vi "G4SubTemplate_Singleton_6x8x6_Init.vi"(0 "reference in":refnum<class "G4SubTemplate_Singleton_6x8x6.lvclass"> caption="This control should only be used when\na sub class is inheriting this class", 5 "error in (no error)":errorcluster) -> (14 "reference out":refnum<class "G4SubTemplate_Singleton_6x8x6.lvclass"> caption="This indicator should only be used when\na sub class is inheriting this class", 19 "error out":errorcluster)   [LabVIEW 2014, in "G4SubTemplate_Singleton_6x8x6.lvclass"]
uses:
  <resource>/Framework/Providers/Open_GDS/ClassProviders/Provider_EndevoGOOP400/Templates/G4SubTemplate_Singleton_6x8x6/G4SubTemplate_Singleton_6x8x6.lvclass
  <resource>/Framework/Providers/Open_GDS/ClassProviders/Provider_EndevoGOOP400/Templates/G4BaseTemplate_Singleton_6x8x6/G4BaseTemplate_Singleton_6x8x6.lvclass
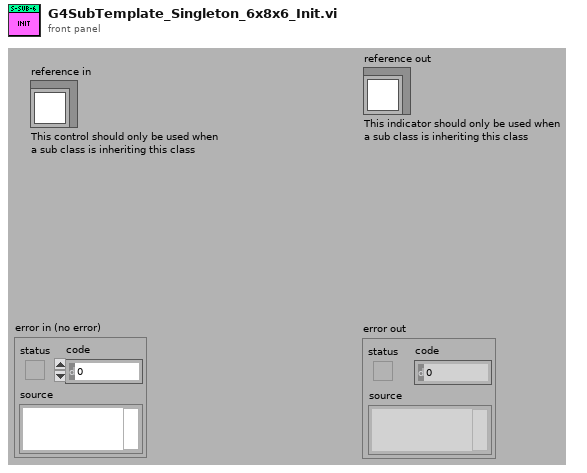
[diagram p1: front panel]
types:
  T1 = typedef "G4SubTemplate_Singleton_6x8x6.lvclass/ObjectAttributes.ctl" = cluster{"Attribute1":dbl}
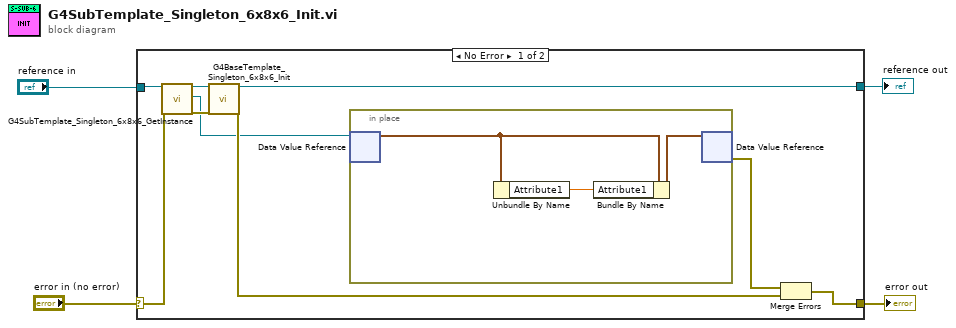
[diagram p0: block diagram]
diagram:
  n1 = case shown="No Error" "error in (no error)" {
    selector: "error in (no error)" -> [w10 w18]
    tunnel: [w12 w18] -> w3
    tunnel: "reference in" -> [w8 w17]
    tunnel: [w7 w17] -> w1
    frame No Error {
      n2 = call <resource>:"G4SubTemplate_Singleton_6x8x6_GetInstance.vi"("reference in"=w8, "error in (no error)"=w10) -> ("reference out"=w6:refnum<class "G4SubTemplate_Singleton_6x8x6.lvclass">, "DVRRefOut"=w5:refnum<data-value>, "error out"=w9:errorcluster)  [unwired: 13 in, 2 out]
      n3 = call <resource>:"G4BaseTemplate_Singleton_6x8x6_Init.vi"("reference in"=w6, "error in (no error)"=w9) -> ("reference out"=w7:refnum<class "G4SubTemplate_Singleton_6x8x6.lvclass">, "error out"=w11:errorcluster)  [unwired: 16 in]
      n4 = in-place {
        n5 = in-place-dvr #1(w5) -> (w15:T1)  [unwired: 1 out]
        n6 = Unbundle By Name(w15) -> ("Attribute1"=w14:dbl)
        n7 = Bundle By Name(cluster=w15, "Attribute1"=w14) -> (w16:T1)
        n8 = in-place-dvr #1(w16) -> (w13:errorcluster)  [unwired: 1 out]
      }
      n9 = Merge Errors(w13, w11) -> (w12:errorcluster)
    }
    frame Error {
    }
  }
  "error out" <- w3
  "reference out" <- w1
